vi "AO Post Step Type.vi"(8 "error in (no error)":errorcluster, 9 "AOWrite":T1, 10 "Socket No":u16=1, 11 "NI Waveform Output in":refnum<class "NI Waveform Output.lvclass">) -> (0 "error out":errorcluster, 2 "PhysicalChannel":string[](array[string]), 3 "NI Waveform Output out":refnum<class "NI Waveform Output.lvclass">)   [LabVIEW 2023, in "HardwareAbstractionLayer_LVOOP.lvlib" / "NI Waveform Output.lvclass"]
doc: "Set attributes of waveform genaration for all selcted channel In Database"
uses:
  NI Waveform Output.lvclass
  NI Waveform Output.lvclass/NI Waveform Output.ctl
  <vilib>/DAQmx/write.llb/DAQmx Write (Analog 1D Wfm NChan NSamp).vi
  <vilib>/DAQmx/miscellaneous.llb/DAQmx Fill In Error Info.vi
  Database/Database.lvclass
  <vilib>/measure/NI_MABase.lvlib
  <resource>/objmgr/daqmx.rc
panel:
  out "Waveform Graph":waveform(dbl)[](graph)=[{"t0"=timestamp(0 s since 1904-01-01), "dt"=0.001, "Y"=[]}]
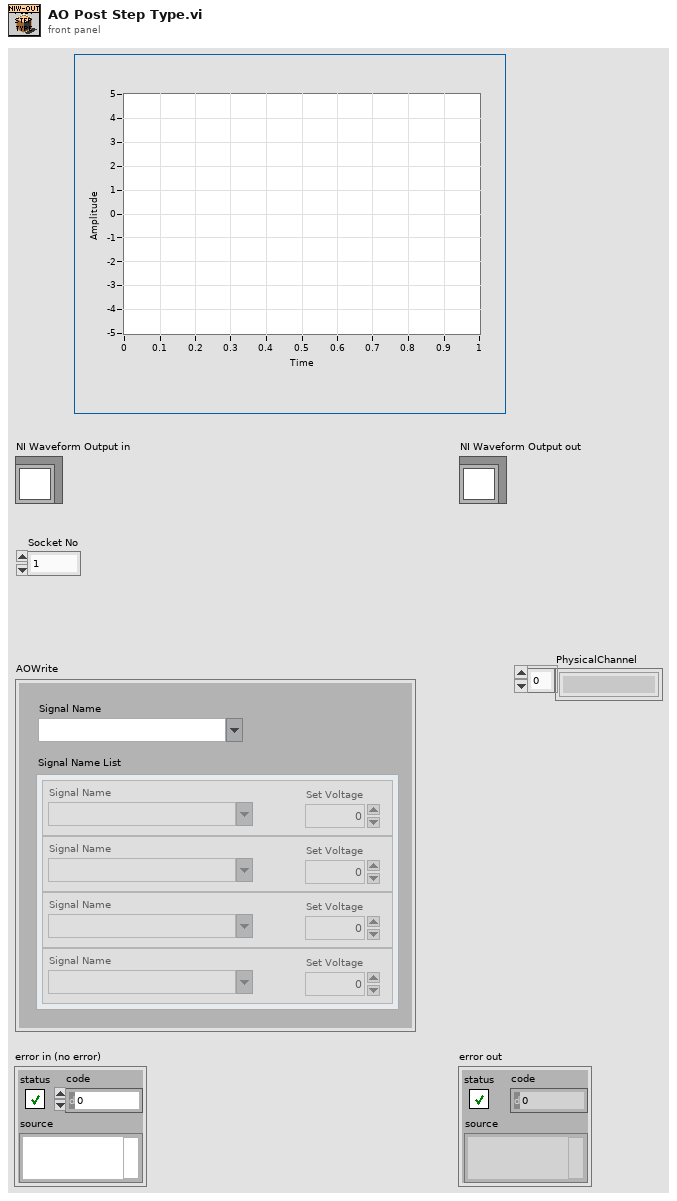
[diagram p1: front panel]
types:
  T1 = cluster{"Signal Name":string, "Signal Name List":cluster{"Signal Name":string, "Set Voltage":dbl}[]}
  T2 = cluster{"table":string, "condition":string, "columns":string[]}
  T3 = cluster{"Waveform Type":u16, "Amplitude":dbl, "Frequency":dbl, "phase":dbl}
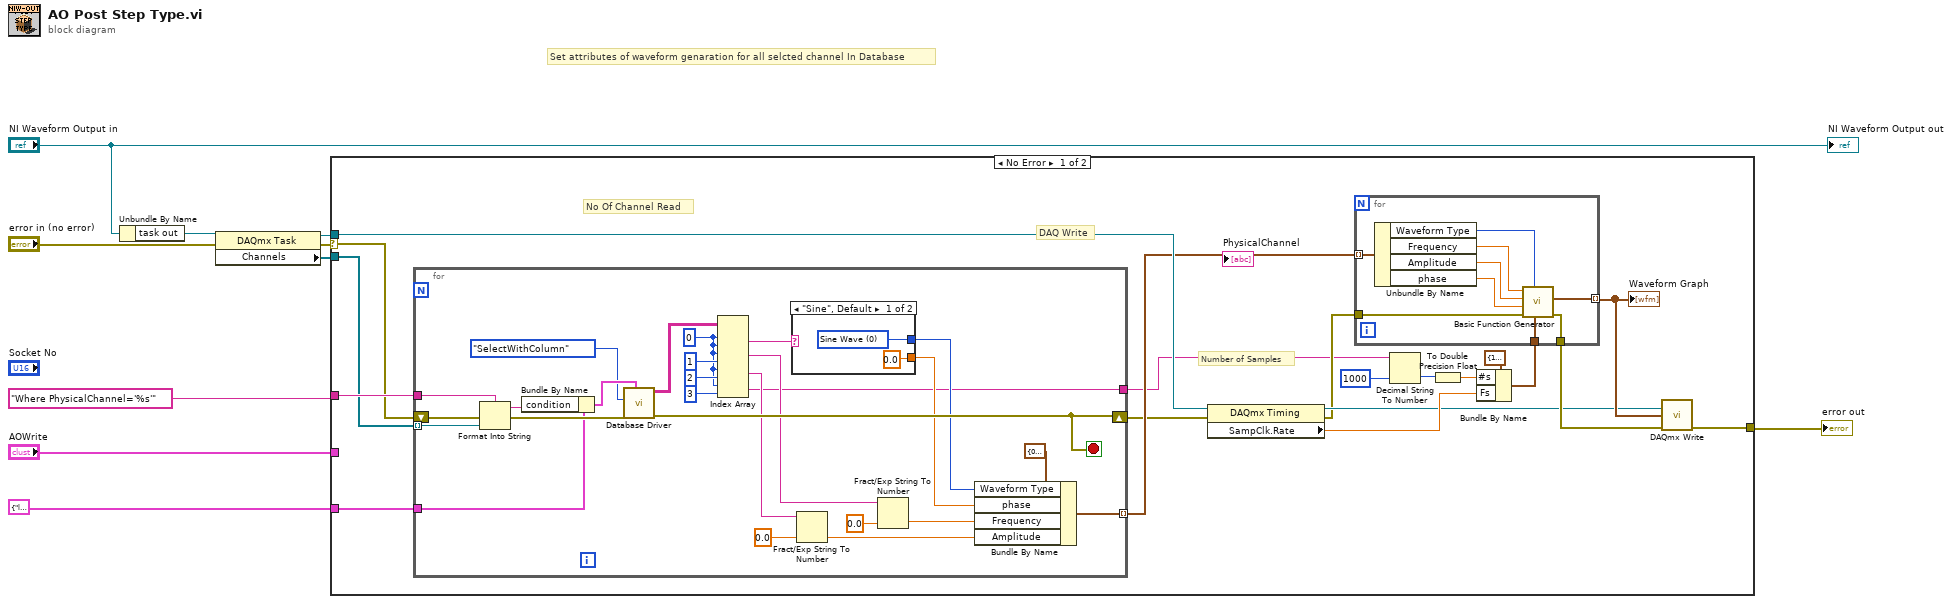
[diagram p0: block diagram]
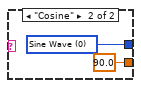
[diagram p2: hidden frame]
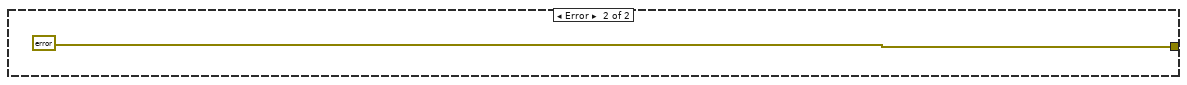
[diagram p3: hidden frame]
diagram:
  # "Set attributes of waveform genaration for all selcted channel In Database"
  n1 = Unbundle By Name("NI Waveform Output in") -> ("task out"=w7:refnum<k21>)
  n2 = property class="DAQmx Task"(reference=w7, error in="error in (no error)") -> (reference out=w3:refnum<k21>, error out=w4:errorcluster, "Channels"=w5:refnum<k21>[])
  n3 = case shown="No Error" w4 {
    selector: w4 -> [w18 _]
    tunnel: [w17 errorcluster {"status"=TRUE, "code"=0, "source"="Analog Waveform generation is errored. Please check the task"} ("error out")] -> w8
    tunnel: "AOWrite" -> [_ _]
    tunnel: "Where PhysicalChannel='%s'" -> [w29 _]
    tunnel: w5 -> [w11 _]
    tunnel: w3 -> [w23 _]
    tunnel: T2 {"table"="ltt.daq_configuration", "condition"="", "columns"=["WaveformType", "Frequency", "Amplitude", "SampleRate"]} ("SQLTableData") -> [w16 _]
    frame No Error {
      # "Number of Samples"
      # "No Of Channel Read"
      # "DAQ Write"
      n4 = for {
        tunnel: w29 -> [w55]
        shift-right: [w46] -> w12
        shift-left: w18 -> [w52]
        tunnel: w11 -> [w34] mode=indexing
        tunnel: [w48] -> w19 mode=indexing
        tunnel: w16 -> [w45]
        tunnel: [w30] -> w13
        stop <- w46 stop-if-true
        w35 = 0 ("disabled index (col)")
        n5 = Format Into String(format string=w55, error in=w52, w34) -> (resulting string=w54:string, error out=w51:errorcluster)  [unwired: 1 in]
        n6 = Bundle By Name(cluster=w45, "condition"=w54) -> (w53:T2)
        n7 = call "Database Driver.vi"("SQLTableData"=w53, "error in"=w51, "Select"=enum16{"SelectWithQuery", "SelectWithColumn"}."SelectWithColumn") -> ("error out"=w46:errorcluster, "data"=w50:string[][])  [unwired: 5 in, 2 out]
        n8 = Index Array(array=w50, index (row) #1=w35, index (col) #1=w35, index (row) #2=w35, index (col) #2=1 ("index (col)"), index (row) #3=w35, index (col) #3=2 ("disabled index (col)"), index (row) #4=w35, index (col) #4=3 ("disabled index (col)")) -> (element #1=w33:string, element #2=w32:string, element #3=w31:string, element #4=w30:string)
        n9 = case shown="\"Sine\", Default" w33 {
          tunnel: [w57 w59] -> w41
          tunnel: [0.0 ("phase") 90.0 ("phase")] -> w40
          frame "Sine", Default {
            w57 = u16 0 items=["Sine Wave", "Triangle Wave", "Square Wave", "Sawtooth Wave"] ("Waveform Type")
          }
          frame "Cosine" {
            w59 = u16 0 items=["Sine Wave", "Triangle Wave", "Square Wave", "Sawtooth Wave"] ("Waveform Type")
          }
        }
        n10 = Fract/Exp String To Number(string=w31, default (0 dbl)=0.0 ("Amplitude")) -> (number=w36:dbl)  [unwired: 2 in, 1 out]
        n11 = Fract/Exp String To Number(string=w32, default (0 dbl)=0.0 ("Frequency")) -> (number=w38:dbl)  [unwired: 2 in, 1 out]
        n12 = Bundle By Name(cluster=T3 {"Waveform Type"=0, "Amplitude"=1.0, "Frequency"=10.0, "phase"=0.0} ("Cluster"), "Waveform Type"=w41, "phase"=w40, "Frequency"=w38, "Amplitude"=w36) -> (w48:T3)
      }
      n13 = property class="DAQmx Timing"(reference=w23, error in=w12) -> (reference out=w21:refnum<k21>, error out=w20:errorcluster, "SampClk.Rate"=w22:dbl)
      n14 = Decimal String To Number(string=w13, default (0L)=1000 ("Number of Samples")) -> (number=w14:i32)  [unwired: 1 in, 1 out]
      n15 = To Double Precision Float(number=w14) -> (double precision float=w24:dbl)
      n16 = Bundle By Name(cluster=cluster{"Fs":dbl, "#s":dbl} {"Fs"=1000.0, "#s"=1000.0} ("sampling info"), "#s"=w24, "Fs"=w22) -> (w27:cluster{"Fs":dbl, "#s":dbl})
      n17 = for {
        tunnel: w27 -> [w68]
        tunnel: [w67] -> w26
        tunnel: w19 -> [w66] mode=indexing
        tunnel: [w62] -> w25 mode=indexing
        tunnel: w20 -> [w61]
        n18 = Unbundle By Name(w66) -> ("Waveform Type"=w65:u16, "Frequency"=w64:dbl, "Amplitude"=w63:dbl, "phase"=w60:dbl)
        n19 = call <vilib>:"Basic Function Generator.vi"("sampling info"=w68, "signal type"=w65, "error in (no error)"=w61, "phase"=w60, "amplitude"=w63, "frequency"=w64) -> ("error out"=w67:errorcluster, "signal out"=w62:waveform(dbl))  [unwired: 3 in, 1 out]
      }
      "Waveform Graph" <- w25
      n20 = call-poly <vilib>:"DAQmx Write.vi"("task/channels in"=w21, "data"=w25, "error in"=w26) -> ("error out"=w17:errorcluster)  [unwired: 10 in, 2 out]
    }
    frame Error {
    }
  }
  "error out" <- w8
  "NI Waveform Output out" <- "NI Waveform Output in"
